vi "CW_enable.vi"(2 "Timeout (ms)":i32=40000000, 3 "connection ID in":refnum<k5>) -> (0 "Timeout (ms) 2":i32=40000000, 1 "connection ID out":refnum<k5>)   [LabVIEW 2016]
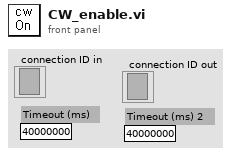
[diagram p1: front panel]
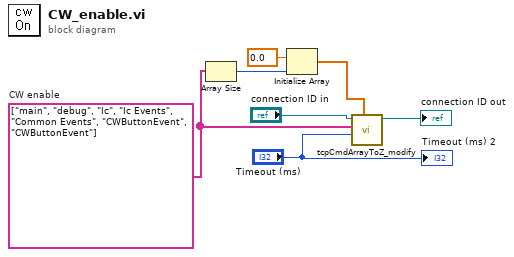
[diagram p0: block diagram]
diagram:
  w4 = string[] ["main", "debug", "Ic", "Ic Events", "Common Events", "CWButtonEvent", "CWButtonEvent"]  # CW enable
  n1 = Array Size(array=w4) -> (size(s)=w7:i32)
  n2 = Initialize Array(0.0 ("element"), w7) -> (w5:dbl[])
  n3 = call "tcpCmdArrayToZ_modify.vi"("Delay (sec)"=w5, "Timeout (ms)"="Timeout (ms)", "Command array"=w4, "connection ID in"="connection ID in") -> ("connection ID out"=→"connection ID out":refnum<k5>)  [unwired: 3 in, 4 out]
  "Timeout (ms) 2" <- "Timeout (ms)"
